vi "VNA_RESET-CLS.vi"(8 "error in":errorcluster {"code" format="%.0x"}, 11 "Session In":refnum<visa-resource-name>="GPIB0::16::INSTR") -> (0 "error out":errorcluster {"code" format="%.0x"}, 3 "Session Out":refnum<visa-resource-name>)   [LabVIEW 2018]
panel:
  in  "cmd":string="*RST;*CLS"
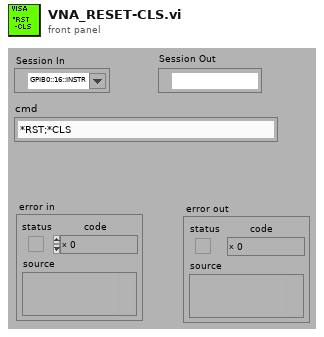
[diagram p1: front panel]
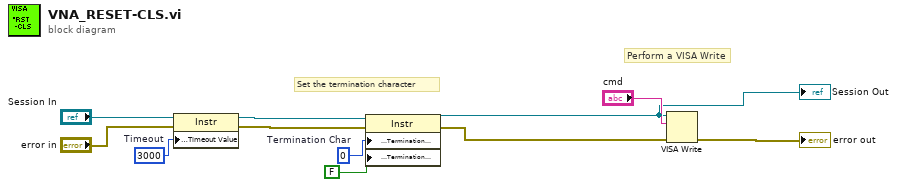
[diagram p0: block diagram]
diagram:
  w6 = u8 0  # Termination Char
  w11 = u32 3000  # Timeout
  # "Perform a VISA Write"
  # "Set the termination character"
  n1 = property class="Instr"(reference="Session In", error in="error in", "General Settings:Timeout Value"=w11) -> (reference out=w5:refnum<visa-resource-name>, error out=w8:errorcluster)
  n2 = property class="Instr"(reference=w5, error in=w8, "Message Based Settings:Termination Character"=w6, "Message Based Settings:Termination Character Enable"=FALSE ("enable")) -> (reference out=w1:refnum<visa-resource-name>, error out=w7:errorcluster)
  "Session Out" <- w1
  n3 = VISA Write(VISA resource name=w1, write buffer="cmd", error in (no error)=w7) -> (error out=→"error out":errorcluster)  [unwired: 2 out]
